vi "matrix_matrix_multiply_FXP_32_16.vi"(1 "p":i32, 3 "n":i32, 4 "m":i32, 5 "B":fxp<+/-,32,16>[](array[numeric]), 6 "A":fxp<+/-,32,16>[](array[numeric])) -> (0 "C":fxp<+/-,32,16>[](array[numeric]))   [LabVIEW 2020]
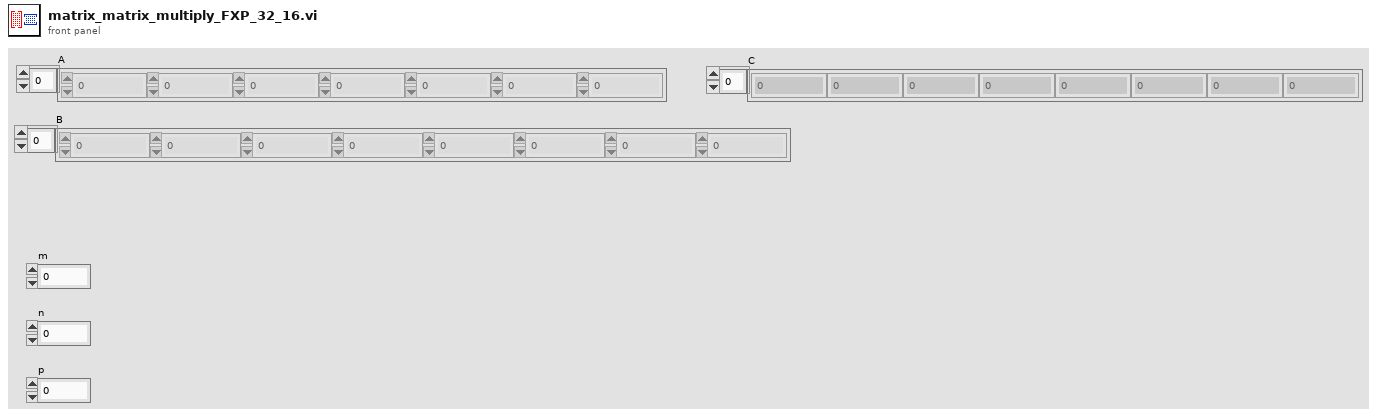
[diagram p1: front panel]
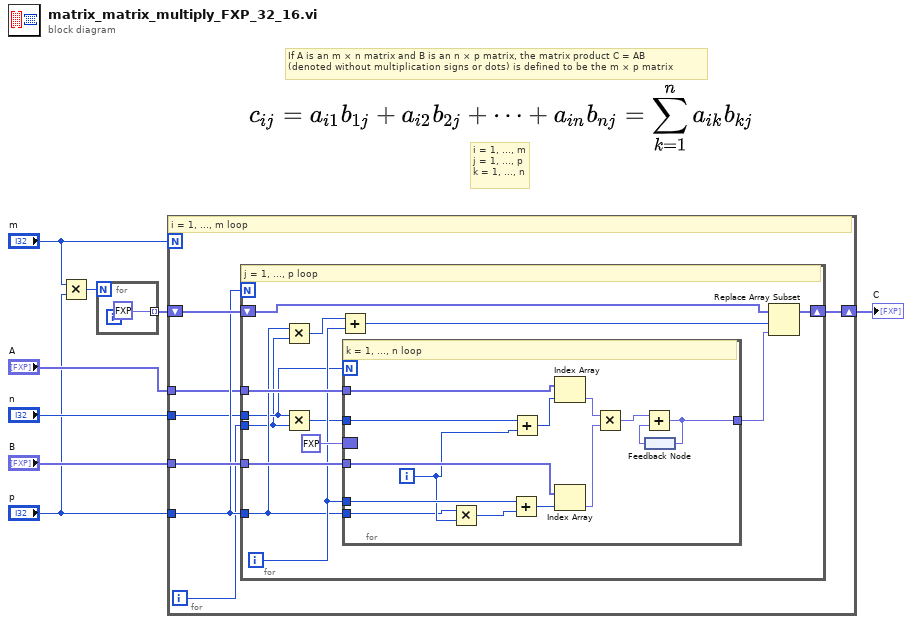
[diagram p0: block diagram]
diagram:
  # "If A is an m × n matrix and B is an n × p matrix, the matrix product C = AB \n(denoted without multiplication signs or dots) is defined to be the m × p matrix"
  # "i = 1, ..., m\nj = 1, ..., p\nk = 1, ..., n"
  n1 = Multiply(x="m", y="p") -> (x*y=w4:i32)
  n2 = for {
    N: w4 -> [_]
    tunnel: [fxp<+/-,32,16> 0.0] -> w1 mode=indexing
  }
  n3 = for {
    N: "m" -> [_]
    tunnel: "B" -> [w16]
    tunnel: "p" -> [w13]
    tunnel: "A" -> [w12]
    tunnel: "n" -> [w11]
    shift-right: [w14] -> w6
    shift-left: w1 -> [w15]
    i -> [w10]
    # "i = 1, ..., m loop"
    n4 = for {
      N: w13 -> [_]
      tunnel: w12 -> [w29]
      tunnel: w16 -> [w28]
      tunnel: w13 -> [w19]
      shift-right: [w25] -> w14
      shift-left: w15 -> [w26]
      tunnel: w11 -> [w18]
      tunnel: w10 -> [w17]
      i -> [w22]
      # "j = 1, ..., p loop"
      n5 = Multiply(x=w19, y=w17) -> (x*y=w21:i32)
      n6 = Multiply(x=w18, y=w17) -> (x*y=w20:i32)
      n7 = Add(x=w21, y=w22) -> (x+y=w23:i32)
      n8 = for {
        N: w18 -> [_]
        tunnel: w29 -> [w43]
        tunnel: w20 -> [w30]
        tunnel: w28 -> [w42]
        tunnel: w22 -> [w36]
        tunnel: [w37] -> w24
        tunnel: w19 -> [w34]
        border: fxp<+/-,32,16> 0.0 -> [_]
        i -> [w35]
        # "k = 1, ..., n loop"
        n9 = Multiply(x=w34, y=w35) -> (x*y=w33:i32)
        n10 = Add(x=w36, y=w33) -> (x+y=w32:i32)
        n11 = Add(x=w30, y=w35) -> (x+y=w31:i32)
        n12 = Index Array(array=w43, index=w31) -> (element=w41:fxp<+/-,32,16>)
        n13 = Index Array(array=w42, index=w32) -> (element=w40:fxp<+/-,32,16>)
        n14 = Multiply(x=w41, y=w40) -> (x*y=w39:fxp<+/-,64,32>)
        n15 = feedback #1() -> (w38:fxp<+/-,32,16>)
        n16 = Add(x=w39, y=w38) -> (x+y=w37:fxp<+/-,32,16>)
        n17 = feedback-in #1(w37) -> ()
      }
      n18 = Replace Array Subset(array=w26, new element=w24, index=w23) -> (w25:fxp<+/-,32,16>[])
    }
  }
  "C" <- w6
